vi "TX main.vi"() -> ()   [LabVIEW 2014]
panel:
  out "unsigned byte array":u8[](array[numeric])
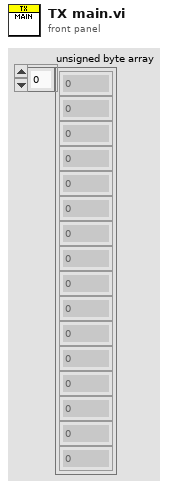
[diagram p1: front panel]
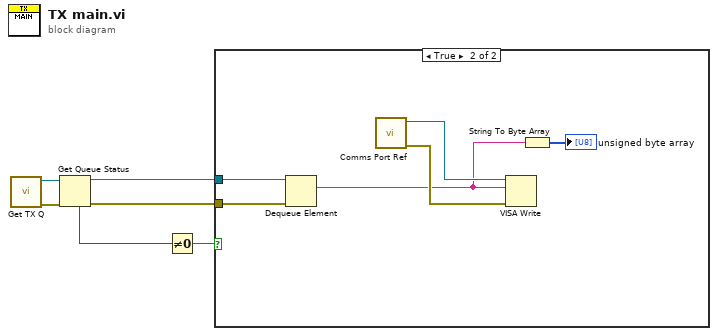
[diagram p0: block diagram]
diagram:
  n1 = call "Get TX Q.vi"() -> ("error out"=w5:errorcluster, "TX Q"=w6:refnum<queue>)  [unwired: 10 in]
  n2 = Get Queue Status(queue=w6, error in (no error)=w5) -> (queue out=w3:refnum<queue>, error out=w2:errorcluster, # elements in queue=w1:i32)  [unwired: 1 in, 5 out]
  n3 = Not Equal To 0?(x=w1) -> (x != 0?=w4:bool)
  n4 = case shown="True" w4 {
    tunnel: w3 -> [_ w12]
    tunnel: w2 -> [_ w11]
    frame False {
    }
    frame True {
      n5 = Dequeue Element(queue=w12, error in (no error)=w11) -> (element=w8:string)  [unwired: 1 in, 3 out]
      n6 = call "Comms Port Ref.vi"() -> ("error out"=w9:errorcluster, "Comms Port Ref"=w10:refnum<visa-resource-name>)  [unwired: 10 in]
      n7 = VISA Write(VISA resource name=w10, write buffer=w8, error in (no error)=w9) -> ()  [unwired: 3 out]
      n8 = String To Byte Array(string=w8) -> (unsigned byte array=→"unsigned byte array":u8[])
    }
  }
